vi "intervalo2.vi"(9 "incremento":dbl, 10 "fin":dbl, 11 "inicio":dbl) -> (2 "Array":dbl[](array[numeric]))   [LabVIEW 2016]
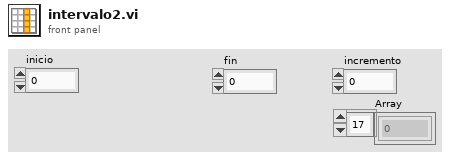
[diagram p1: front panel]
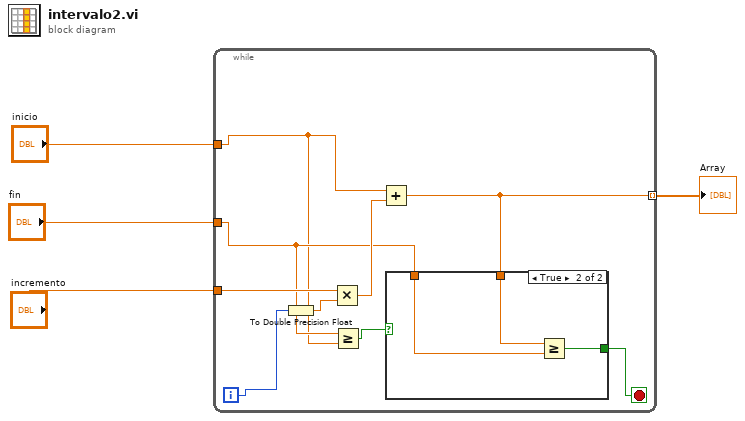
[diagram p0: block diagram]
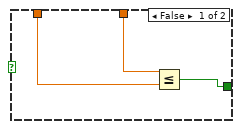
[diagram p2: hidden frame]
diagram:
  n1 = while {
    tunnel: "inicio" -> [w5]
    tunnel: "fin" -> [w6]
    tunnel: "incremento" -> [w13]
    tunnel: [w8] -> w1 mode=indexing
    i -> [w11]
    stop <- w9 stop-if-true
    n2 = To Double Precision Float(number=w11) -> (double precision float=w12:dbl)
    n3 = Multiply(x=w13, y=w12) -> (x*y=w10:dbl)
    n4 = Greater Or Equal?(x=w6, y=w5) -> (x >= y?=w7:bool)
    n5 = Add(x=w5, y=w10) -> (x+y=w8:dbl)
    n6 = case shown="True" w7 {
      tunnel: [w16 w19] -> w9
      tunnel: w8 -> [w15 w18]
      tunnel: w6 -> [w14 w17]
      frame False {
        n7 = Less Or Equal?(x=w15, y=w14) -> (x <= y?=w16:bool)
      }
      frame True {
        n8 = Greater Or Equal?(x=w18, y=w17) -> (x >= y?=w19:bool)
      }
    }
  }
  "Array" <- w1
